vi "plotBoardAndPieces.vi"(8 "error in (no error)":errorcluster, 11 "object in":refnum<class "Board.lvclass">) -> (0 "error out":errorcluster, 3 "object out":refnum<class "Board.lvclass">)   [LabVIEW 2020, in "Board.lvclass"]
uses:
  Board.lvclass
  Pieces/Piece.lvclass/Piece.ctl
  Board.lvclass/Board.ctl
  <vilib>/picture/picture.llb/Draw True-Color Pixmap.vi
  Pieces/Piece.lvclass
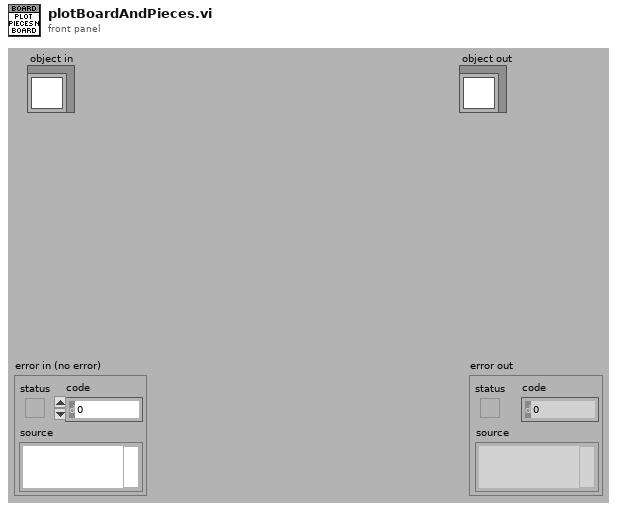
[diagram p1: front panel]
types:
  T1 = typedef "Board.lvclass/pieceMap.ctl" = map{map{string, i32}, refnum<class "Piece.lvclass">}
  T2 = typedef "imagedata.ctl" = cluster{"image type":i32, "image depth":i32, "image":u8[], "mask":u8[], "colors":u32[], "Rectangle":cluster{"left":i16, "top":i16, "right":i16, "bottom":i16}}
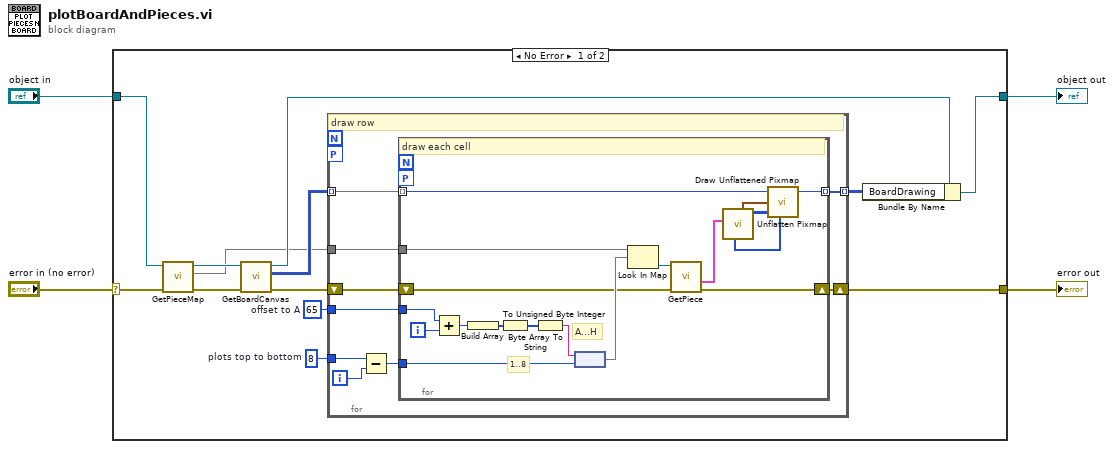
[diagram p0: block diagram]
diagram:
  n1 = case shown="No Error" "error in (no error)" {
    selector: "error in (no error)" -> [w16 w46]
    tunnel: [w13 w46] -> w3
    tunnel: [w17 w45] -> w1
    tunnel: "object in" -> [w14 w45]
    frame No Error {
      w6 = 8  # plots top to bottom
      w7 = 65  # offset to A
      n2 = call "GetPieceMap.vi"("error in (no error)"=w16, "object in"=w14) -> ("error out"=w15:errorcluster, "pieceMap"=w8:T1, "object out"=w11:refnum<class "Board.lvclass">)  [unwired: 6 in, 1 out]
      n3 = call "GetBoardCanvas.vi"("error in (no error)"=w15, "object in"=w11) -> ("error out"=w12:errorcluster, "boardCanvas"=w9:picture[][], "object out"=w10:refnum<class "Board.lvclass">)  [unwired: 7 in]
      n4 = for {
        tunnel: w9 -> [w26] mode=indexing
        tunnel: [w25] -> w5 mode=indexing
        shift-right: [w23] -> w13
        shift-left: w12 -> [w24]
        tunnel: w8 -> [w22]
        tunnel: w7 -> [w21]
        tunnel: w6 -> [w20]
        workers-P: _ -> [_]
        i -> [w19]
        # "draw row"
        n5 = Subtract(x=w20, y=w19) -> (x-y=w18:i32)
        n6 = for {
          tunnel: w26 -> [w44] mode=indexing
          tunnel: [w43] -> w25 mode=indexing
          shift-right: [w27] -> w23
          shift-left: w24 -> [w28]
          tunnel: w22 -> [w36]
          tunnel: w21 -> [w33]
          tunnel: w18 -> [w30]
          workers-P: _ -> [_]
          i -> [w29]
          # "1..8"
          # "A...H"
          # "draw each cell"
          n7 = Add(x=w33, y=w29) -> (x+y=w34:i32)
          n8 = Build Array(w34) -> (w38:i32[])
          n9 = To Unsigned Byte Integer(number=w38) -> (unsigned 8bit integer=w39:u8[])
          n10 = Byte Array To String(unsigned byte array=w39) -> (string=w37:string)
          n11 = node(w37, w30) -> (w35:map{string, i32})
          n12 = Look In Map(map=w36, key=w35) -> (value=w32:refnum<class "Piece.lvclass">)  [unwired: 1 in, 1 out]
          n13 = call "GetPiece.vi"("error in (no error)"=w28, "Piece in"=w32) -> ("error out"=w27:errorcluster, "pieceDrawing"=w31:T2)  [unwired: 5 in, 3 out]
          n14 = call <vilib>:"Unflatten Pixmap.vi"("image data"=w31) -> ("24-bit pixmap"=w42:u32[][], "top left"=w40:cluster{"x":i16, "y":i16}, "mask"=w41:u8[])  [unwired: 4 in, 4 out]
          n15 = call-poly <vilib>:"Draw Unflattened Pixmap.vi"("picture"=w44, "top left point(0, 0)"=w40, "data (RGB format)"=w42, "mask"=w41) -> ("new picture"=w43:picture)  [unwired: 5 in]
        }
      }
      n16 = Bundle By Name(cluster=w10, "BoardDrawing"=w5) -> (w17:refnum<class "Board.lvclass">)
    }
    frame Error {
    }
  }
  "error out" <- w3
  "object out" <- w1
